vi "VISA2NMLAddress.vi"(1 "VISA resource name":refnum<visa-resource-name>) -> (0 "NML Address":string)   [LabVIEW 2020]
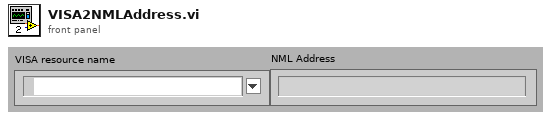
[diagram p1: front panel]
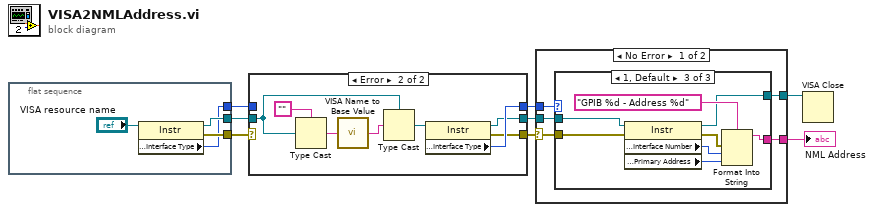
[diagram p0: block diagram]
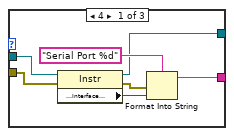
[diagram p2: hidden frame]
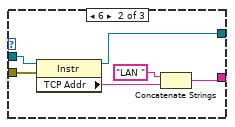
[diagram p3: hidden frame]
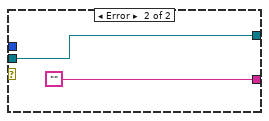
[diagram p4: hidden frame]
diagram:
  n1 = flat-sequence {
    tunnel: [w12] -> w8
    tunnel: [w11] -> w7
    tunnel: [w10] -> w6
    frame #0 {
      n2 = property class="Instr"(reference="VISA resource name") -> (reference out=w12:refnum<visa-resource-name>, error out=w11:errorcluster, "Interface Information:Interface Type"=w10:u16)  [unwired: 1 in]
    }
  }
  n3 = case shown="Error" w7 {
    selector: w7 -> [w14 _]
    tunnel: w8 -> [w15 w18]
    tunnel: w6 -> [w13 _]
    tunnel: [w13 w22] -> w4
    tunnel: [w14 w21] -> w5
    tunnel: [w15 w20] -> w3
    frame No Error {
    }
    frame Error {
      n4 = Type Cast(type="", x=w18) -> (*(type *) &x=w17:string)
      n5 = call "VISA Name to Base Value.vi"("String"=w17) -> ("String 2"=w23:string)
      n6 = Type Cast(type=w18, x=w23) -> (*(type *) &x=w19:refnum<visa-resource-name>)
      n7 = property class="Instr"(reference=w19) -> (reference out=w20:refnum<visa-resource-name>, error out=w21:errorcluster, "Interface Information:Interface Type"=w22:u16)  [unwired: 1 in]
    }
  }
  n8 = case shown="No Error" w5 {
    selector: w5 -> [w25 _]
    tunnel: [w28 ""] -> w1
    tunnel: w4 -> [w27 _]
    tunnel: w3 -> [w26 w50]
    tunnel: [w24 w50] -> w2
    frame No Error {
      n9 = case shown="1, Default" w27 {
        tunnel: [w34 w37 w48] -> w28
        tunnel: w26 -> [w32 w39 w47]
        tunnel: w25 -> [w29 w38 w44]
        tunnel: [w30 w36 w42] -> w24
        frame 4 {
          n10 = property class="Instr"(reference=w32, error in=w29) -> (reference out=w30:refnum<visa-resource-name>, error out=w31:errorcluster, "Interface Information:Interface Number"=w33:u16)
          n11 = Format Into String(format string="Serial Port %d", error in=w31, w33) -> (resulting string=w34:string)  [unwired: 1 in, 1 out]
        }
        frame 6 {
          n12 = property class="Instr"(reference=w39, error in=w38) -> (reference out=w36:refnum<visa-resource-name>, "TCP Addr"=w40:string)  [unwired: 1 out]
          n13 = Concatenate Strings("LAN " ("format string"), w40) -> (w37:string)
        }
        frame 1, Default {
          n14 = property class="Instr"(reference=w47, error in=w44) -> (reference out=w42:refnum<visa-resource-name>, error out=w43:errorcluster, "Interface Information:Interface Number"=w46:u16, "GPIB Settings:Primary Address"=w45:u16)
          n15 = Format Into String(format string="GPIB %d - Address %d", error in=w43, w46, w45) -> (resulting string=w48:string)  [unwired: 1 in, 1 out]
        }
      }
    }
    frame Error {
    }
  }
  "NML Address" <- w1
  n16 = VISA Close(VISA resource name=w2) -> ()  [unwired: 1 in, 1 out]
